vi "Execute Dress right, DRESS!!.vi"(6 "Mouse Position":T1, 8 "User VI Ref":refnum<vi>, 9 "Menu Item Tag Suffix":string, 10 "Remaining Items":refnum<vi>[](array[refnum]), 11 "Affected Items":T2) -> (0 "Fail transaction?":bool)   [LabVIEW 2025]
doc: "This VI is part of a plug-in for modifying the LabVIEW shortcut menus. This is the execute VI which is called when the shortcut menu is chosen by the user. It performs the action of the selected menu item."
uses:
  Dress right, DRESS!!.ctl
  <vilib>/Utility/miscctls.llb/LVPositionTypeDef.ctl
panel:
  out "error out":errorcluster
  # "All controls on this panel except \"Affected Items\" have been locked to prevent accidental edits. Changing the control names or types, other than the elements of the \"Affected Items\" cluster will make the VI unusable as a menu plugin.\n\nSee Context Help for each control for details about its use."
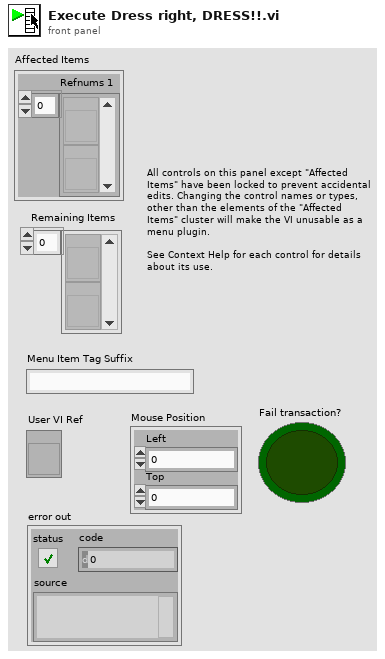
[diagram p1: front panel]
types:
  T1 = typedef "LVPositionTypeDef.ctl" = cluster{"Left":i32, "Top":i32}
  T2 = typedef "Dress right, DRESS!!.ctl" = cluster{"Refnums 1":refnum<vi>[]}
  T3 = enum32{"Top Edges", "Vertical Centers", "Bottom Edges", "Left Edges", "Horizontal Centers", "Right Edges"}
  T4 = enum32{"Top Edges", "Vertical Centers", "Bottom Edges", "Vertical Gap", "Vertical Compress", "Left Edges", "Horizontal Centers", "Right Edges", "Horizontal Gap", "Horizontal Compress"}
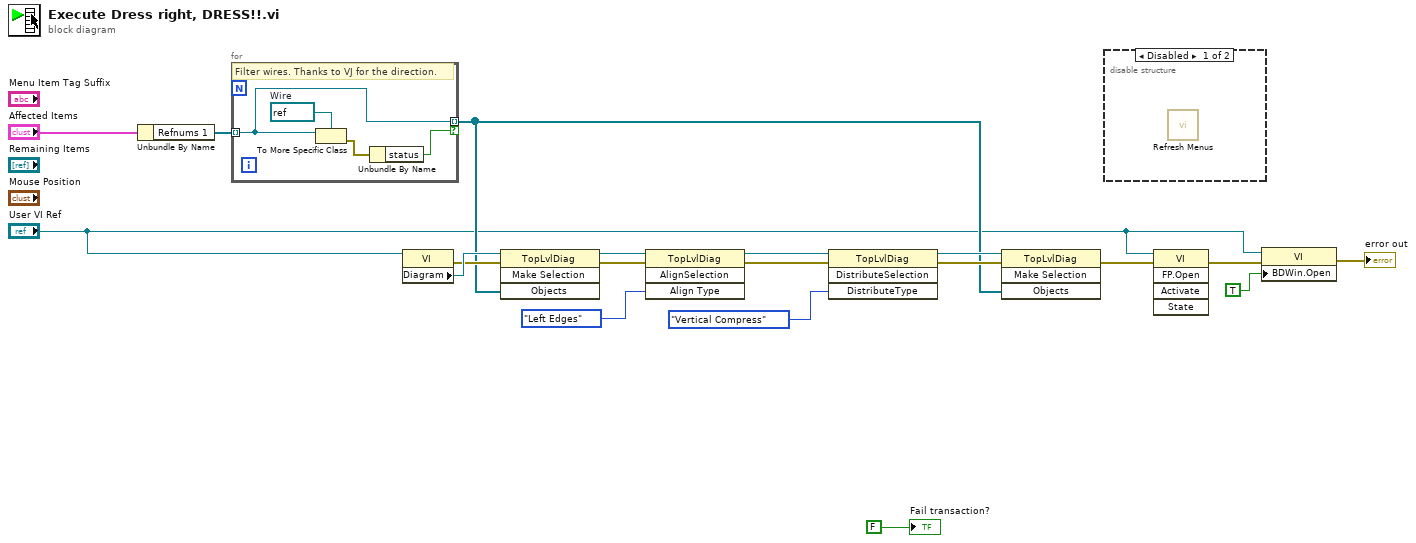
[diagram p0: block diagram]
diagram:
  n1 = Unbundle By Name("Affected Items") -> ("Refnums 1"=w17:refnum<vi>[])
  n2 = for {
    tunnel: w17 -> [w21] mode=indexing
    tunnel: [w21] -> w5 mode=indexing if=w20
    w23 = refnum<vi> refnum  # Wire
    # "Filter wires. Thanks to VJ for the direction."
    n3 = To More Specific Class(target class=w23, reference=w21) -> (error out=w22:errorcluster)  [unwired: 1 in, 1 out]
    n4 = Unbundle By Name(w22) -> ("status"=w20:bool)
  }
  n5 = property class="VI"(reference="User VI Ref") -> (error out=w12:errorcluster, "Diagram"=w13:refnum<vi>)  [unwired: 1 in, 1 out]
  n6 = invoke class="TopLvlDiag" method="Make Selection"(reference=w13, error in=w12, "Objects"=w5) -> (reference out=w11:refnum<vi>, error out=w10:errorcluster)  [unwired: 1 in, 2 out]
  n7 = invoke class="TopLvlDiag" method="AlignSelection"(reference=w11, error in=w10, "Align Type"=T3."Left Edges") -> (reference out=w9:refnum<vi>, error out=w8:errorcluster)  [unwired: 1 in, 2 out]
  n8 = invoke class="TopLvlDiag" method="DistributeSelection"(reference=w9, error in=w8, "DistributeType"=T4."Vertical Compress") -> (reference out=w7:refnum<vi>, error out=w6:errorcluster)  [unwired: 1 in, 2 out]
  n9 = invoke class="TopLvlDiag" method="Make Selection"(reference=w7, error in=w6, "Objects"=w5) -> (error out=w3:errorcluster)  [unwired: 1 in, 3 out]
  n10 = disable-structure shown="Disabled" {
    frame Disabled {
      n11 = call <resource>:"Refresh Menus.vi"() -> ()  [unwired: 12 in]
    }
    frame Enabled {
    }
  }
  n12 = invoke class="VI" method="FP.Open"(reference="User VI Ref", error in=w3) -> (error out=w2:errorcluster)  [unwired: 3 in, 4 out]
  n13 = property class="VI"(reference="User VI Ref", error in=w2, "BDWin.Open"=TRUE ("Block Diagram Window:Open")) -> (error out=→"error out":errorcluster)  [unwired: 1 out]
  "Fail transaction?" <- FALSE ("Fail transaction?")
